vi "algo.configuration.vi"(11 "algo.data.in":T1={"next.state"=enum."Wait.for.Command", "saved.state"=enum."Wait.for.Command", "scratch"={"i"=0, "n"=0, "start.addr"=0, "first.call?"=FALSE, "j"=0, "o"=0, "k"=0, "p"=0, "just.write"=FALSE, "orderId "=0, "dir"=0}, "mode"=enum."Get.Symbol", "cmd.mem.watchlist"={"read.request"=FALSE, "read.addr"=0, "read.ready"=FALSE, "val.watchlist.read"={"symbol"=0, "buy.start.addr"=0, "buy.size"=0, "buy.slots"=0, "sell.start.addr"=0, "sell.size"=0, "sell.slots"=0, "min.ask"=0, "max.bid"=0}, "write.request"=FALSE, "write.addr"=0, "val.watchlist.write"={"symbol"=0, "buy.start.addr"=0, "buy.size"=0, "buy.slots"=0, "sell.start.addr"=0, "sell.size"=0, "sell.slots"=0, "min.ask"=0, "max.bid"=0}}, "cmd.mem.orders"={"read.addr"=0, "read.request"=FALSE, "read.ready"=FALSE, "write.addr"=0, "write.request"=FALSE, "read.data"={"OrderId"=0, "Price"=0, "Quantity"=0}, "write.data"={"OrderId"=0, "Price"=0, "Quantity"=0}}, "cmd.state"={"write.to.state"=FALSE, "val.state"=[0, 0, 0, 0]}, "cmd.debug"={"write.to.debug"=FALSE, "val.debug"=[0, 0]}, "stats"={"min.ask"=0, "max.bid"=0, "price"=0, "quantity"=0, "execution"=FALSE}, "orderbook.command"={"type"=enum."AddOrder", "side"=0, "orderId "=0, "quantity"=0, "symbol"=0, "price"=0, "executed.qty"=0, "canceled.qty"=0, "remaining.qty"=0, "seconds"=0, "nanoseconds"=0, "Add"=FALSE, "Edit"=FALSE, "Remove"=FALSE}, "time"={"last"=0, "since"=0}, "watchlist.size"=0, "active.watchlist"={"item"={"symbol"=0, "buy.start.addr"=0, "buy.size"=0, "buy.slots"=0, "sell.start.addr"=0, "sell.size"=0, "sell.slots"=0, "min.ask"=0, "max.bid"=0}, "index"=0}, "active.order"={"buy"=FALSE, "sell"=FALSE, "addr"=0, "size"=0, "slots"=0, "index"=0}} {"active.watchlist"."item"."symbol" format="%.0x"; "cmd.mem.orders"."write.data"."OrderId" format="%.0x"; "cmd.mem.orders"."read.data"."OrderId" format="%.0x"; "cmd.mem.watchlist"."val.watchlist.write"."symbol" format="%.0x"; "cmd.mem.watchlist"."val.watchlist.read"."symbol" format="%.0x"}) -> (0 "Ready.for.OrderBook.Command.Input":bool, 3 "algo.data.out":T1={"next.state"=enum."Wait.for.Command", "saved.state"=enum."Wait.for.Command", "scratch"={"i"=0, "n"=0, "start.addr"=0, "first.call?"=FALSE, "j"=0, "o"=0, "k"=0, "p"=0, "just.write"=FALSE, "orderId "=0, "dir"=0}, "mode"=enum."Get.Symbol", "cmd.mem.watchlist"={"read.request"=FALSE, "read.addr"=0, "read.ready"=FALSE, "val.watchlist.read"={"symbol"=0, "buy.start.addr"=0, "buy.size"=0, "buy.slots"=0, "sell.start.addr"=0, "sell.size"=0, "sell.slots"=0, "min.ask"=0, "max.bid"=0}, "write.request"=FALSE, "write.addr"=0, "val.watchlist.write"={"symbol"=0, "buy.start.addr"=0, "buy.size"=0, "buy.slots"=0, "sell.start.addr"=0, "sell.size"=0, "sell.slots"=0, "min.ask"=0, "max.bid"=0}}, "cmd.mem.orders"={"read.addr"=0, "read.request"=FALSE, "read.ready"=FALSE, "write.addr"=0, "write.request"=FALSE, "read.data"={"OrderId"=0, "Price"=0, "Quantity"=0}, "write.data"={"OrderId"=0, "Price"=0, "Quantity"=0}}, "cmd.state"={"write.to.state"=FALSE, "val.state"=[0, 0, 0, 0]}, "cmd.debug"={"write.to.debug"=FALSE, "val.debug"=[0, 0]}, "stats"={"min.ask"=0, "max.bid"=0, "price"=0, "quantity"=0, "execution"=FALSE}, "orderbook.command"={"type"=enum."AddOrder", "side"=0, "orderId "=0, "quantity"=0, "symbol"=0, "price"=0, "executed.qty"=0, "canceled.qty"=0, "remaining.qty"=0, "seconds"=0, "nanoseconds"=0, "Add"=FALSE, "Edit"=FALSE, "Remove"=FALSE}, "time"={"last"=0, "since"=0}, "watchlist.size"=0, "active.watchlist"={"item"={"symbol"=0, "buy.start.addr"=0, "buy.size"=0, "buy.slots"=0, "sell.start.addr"=0, "sell.size"=0, "sell.slots"=0, "min.ask"=0, "max.bid"=0}, "index"=0}, "active.order"={"buy"=FALSE, "sell"=FALSE, "addr"=0, "size"=0, "slots"=0, "index"=0}} {"active.watchlist"."item"."symbol" format="%.0x"; "cmd.mem.orders"."write.data"."OrderId" format="%.0x"; "cmd.mem.orders"."read.data"."OrderId" format="%.0x"; "cmd.mem.watchlist"."val.watchlist.write"."symbol" format="%.0x"; "cmd.mem.watchlist"."val.watchlist.read"."symbol" format="%.0x"})   [LabVIEW 2020]
uses:
  <vilib>/rvi/DataTransferAndStorage/Container/XNode/niFpgaContainer.xnode
  types/algo.states.ctl
  <vilib>/rvi/FIFO/Fifo_Resource/nirvififoEmulationRead.vi
  types/algo.scratch.ctl
  types/algo.mode.ctl
  types/algo.val.watchlist.ctl
  types/algo.cmd.mem.watchlist.ctl
  types/algo.cmd.mem.orders.ctl
  types/algo.val.state.ctl
  types/algo.cmd.state.ctl
  types/algo.val.debug.ctl
  types/algo.cmd.debug.ctl
  types/algo.stats.ctl
  common/orderbook.command.type.ctl
  common/orderbook.command.ctl
  types/algo.time.ctl
  algo.data.ctl
  types/algo.val.order.ctl
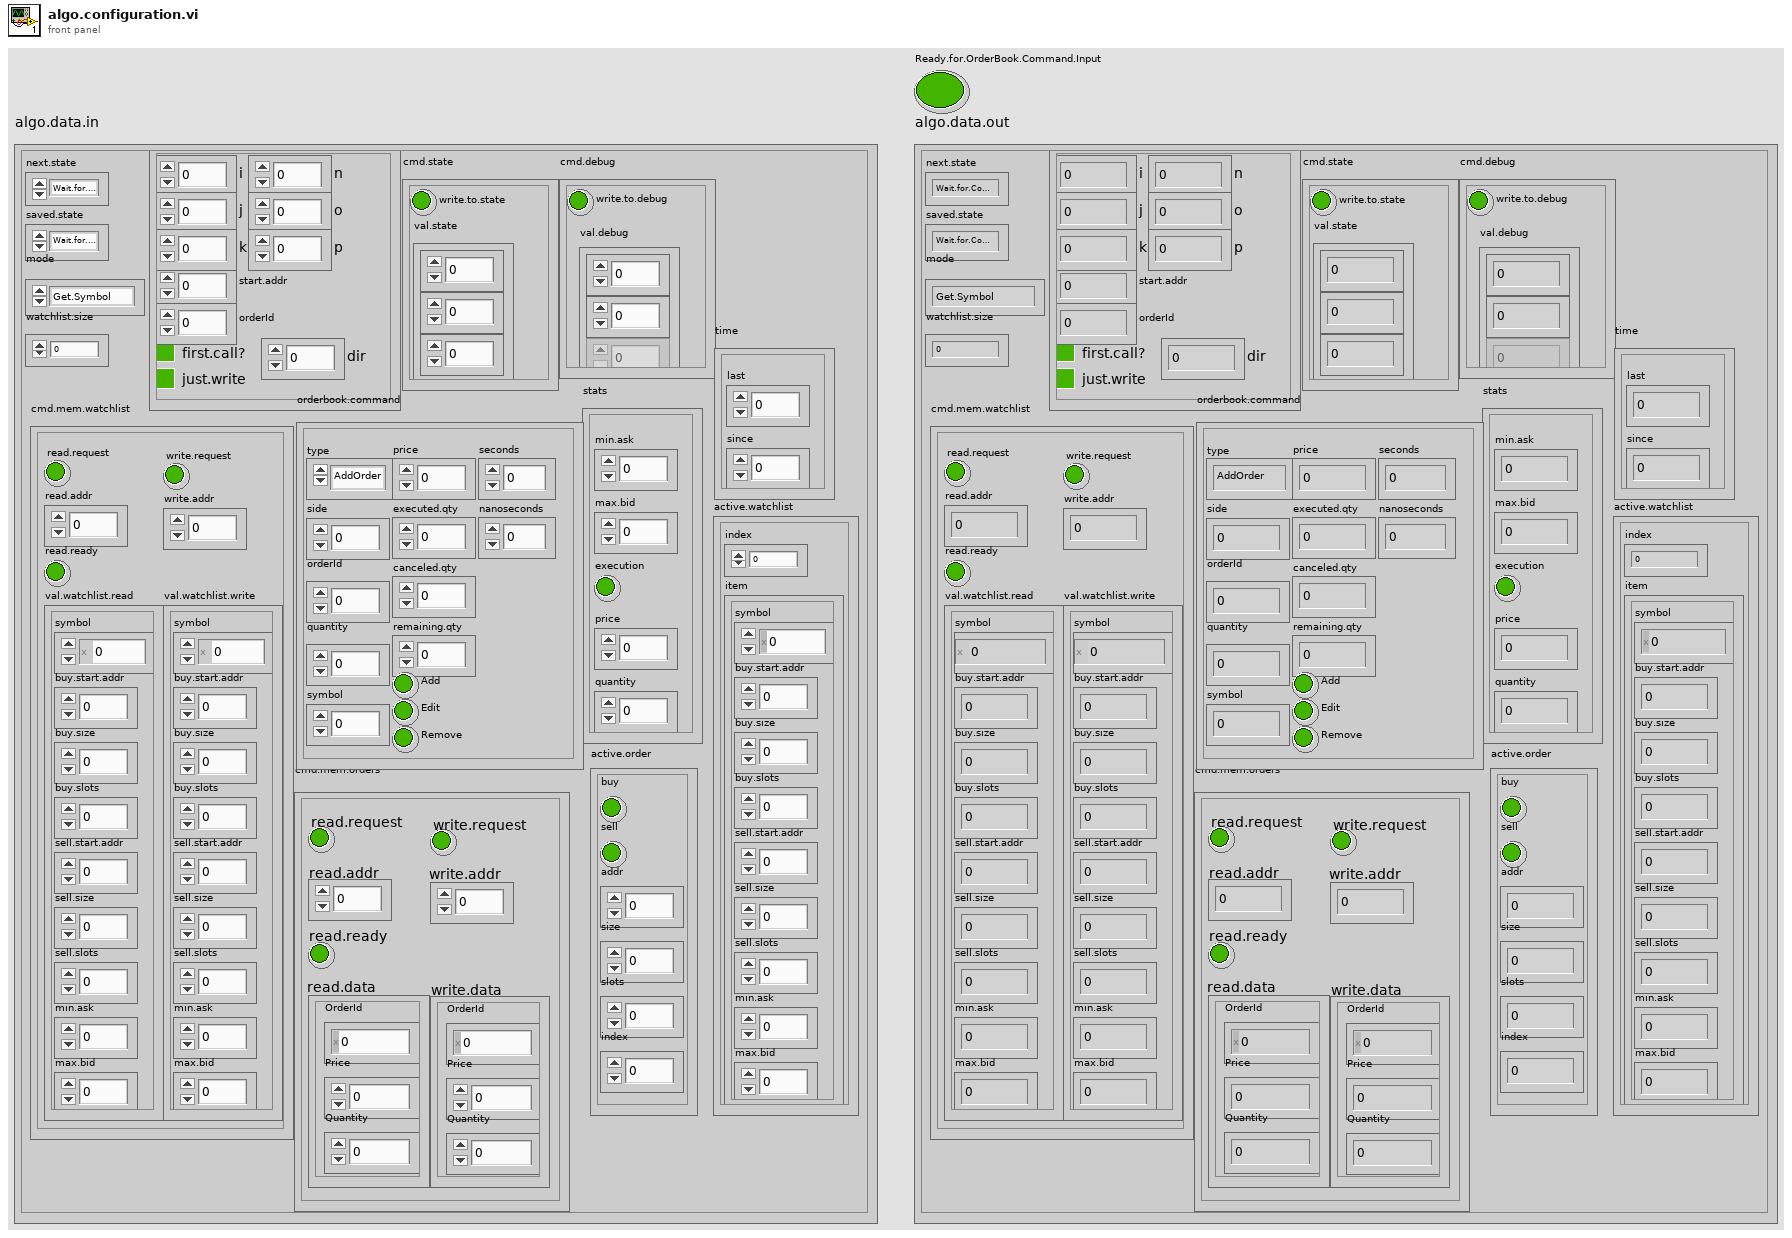
[diagram p1: front panel]
types:
  T1 = typedef "algo.data.ctl" = cluster{"next.state":T2, "saved.state":T2, "scratch":T3, "mode":T4, "cmd.mem.watchlist":T5, "cmd.mem.orders":T7, "cmd.state":T9, "cmd.debug":T11, "stats":T13, "orderbook.command":T14, "time":T16, "watchlist.size":u64, "active.watchlist":cluster{"item":T6, "index":u64}, "active.order":cluster{"buy":bool, "sell":bool, "addr":i16, "size":i16, "slots":i16, "index":i16}}
  T2 = typedef "algo.states.ctl" = enum16{"Noop", "Reset", "Configuration", "Debug", "Get.State", "Wait.for.Command", "Process.Command"}
  T3 = typedef "algo.scratch.ctl" = cluster{"i":u64, "n":u64, "start.addr":u16, "first.call?":bool, "j":u64, "o":u64, "k":u64, "p":u64, "just.write":bool, "orderId ":u64, "dir":i8}
  T4 = typedef "algo.mode.ctl" = enum16{"watchlist.iter", "order.buy.iter", "order.sell.iter", "Get.Symbol", "Search", "Shift"}
  T5 = typedef "algo.cmd.mem.watchlist.ctl" = cluster{"read.request":bool, "read.addr":u16, "read.ready":bool, "val.watchlist.read":T6, "write.request":bool, "write.addr":u16, "val.watchlist.write":T6}
  T6 = typedef "algo.val.watchlist.ctl" = cluster{"symbol":u64, "buy.start.addr":u16, "buy.size":u16, "buy.slots":u16, "sell.start.addr":u16, "sell.size":u16, "sell.slots":u16, "min.ask":u64, "max.bid":u64}
  T7 = typedef "algo.cmd.mem.orders.ctl" = cluster{"read.addr":u16, "read.request":bool, "read.ready":bool, "write.addr":u16, "write.request":bool, "read.data":T8, "write.data":T8}
  T8 = typedef "algo.val.order.ctl" = cluster{"OrderId":u64, "Price":u64, "Quantity":u32}
  T9 = typedef "algo.cmd.state.ctl" = cluster{"write.to.state":bool, "val.state":T10}
  T10 = typedef "algo.val.state.ctl" = u64[]
  T11 = typedef "algo.cmd.debug.ctl" = cluster{"write.to.debug":bool, "val.debug":T12}
  T12 = typedef "algo.val.debug.ctl" = u64[]
  T13 = typedef "algo.stats.ctl" = cluster{"min.ask":u32, "max.bid":u32, "price":u32, "quantity":u32, "execution":bool}
  T14 = typedef "orderbook.command.ctl" = cluster{"type":T15, "side":u8, "orderId ":u64, "quantity":u32, "symbol":u64, "price":u64, "executed.qty":u32, "canceled.qty":u32, "remaining.qty":u32, "seconds":u64, "nanoseconds":u64, "Add":bool, "Edit":bool, "Remove":bool}
  T15 = typedef "orderbook.command.type.ctl" = enum8{"Time", "AddOrder", "OrderExecuted", "OrderExecutedAtPrice", "ReduceSize", "ModifyOrder", "DeleteOrder", "Get.Everything", "Get.All.Orders", "Get.Top"}
  T16 = typedef "algo.time.ctl" = cluster{"last":u32, "since":u32}
  T17 = cluster{"symbol":u64, "buy.start.addr":u16, "buy.size":u16, "buy.slots":u16, "sell.start.addr":u16, "sell.size":u16, "sell.slots":u16, "min.ask":u64, "max.bid":u64}
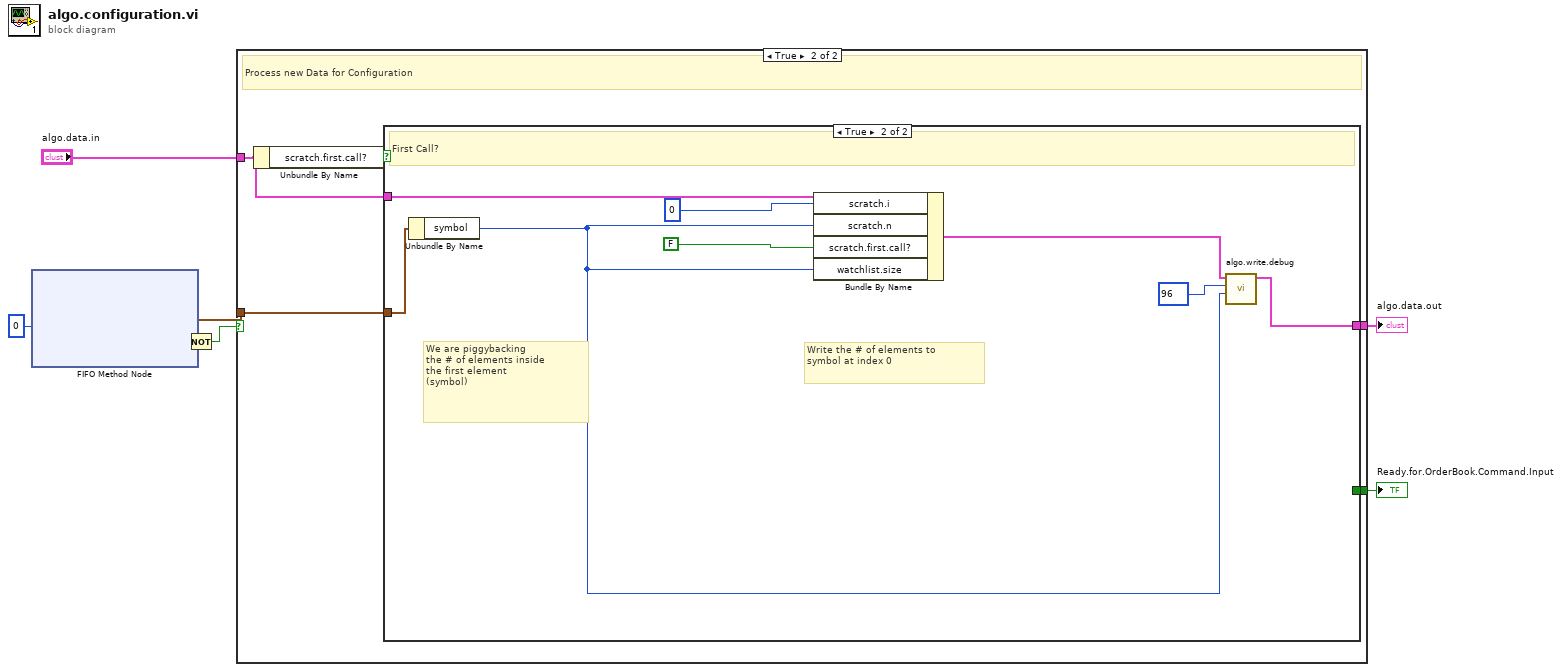
[diagram p0: block diagram]
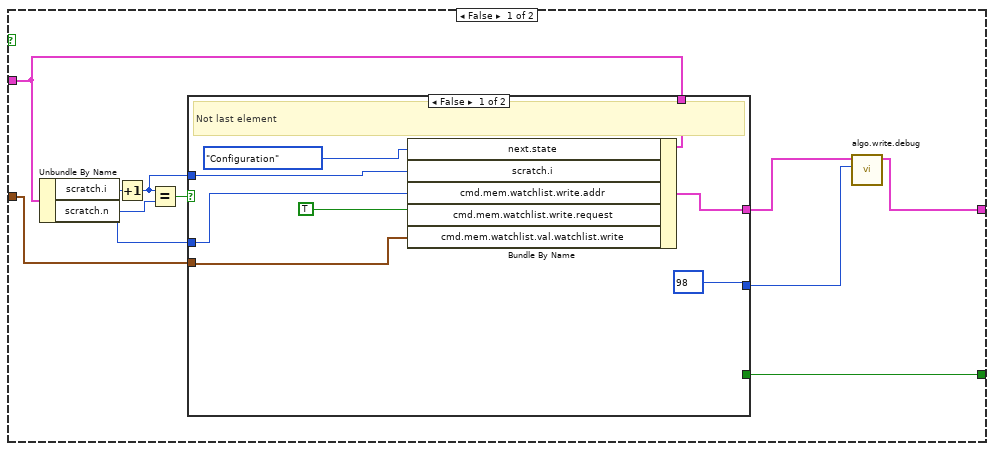
[diagram p3: hidden frame]
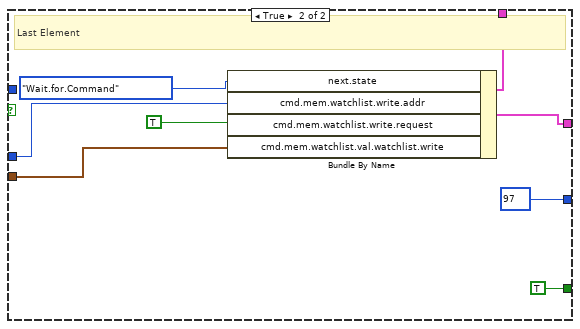
[diagram p4: hidden frame]
diagram:
  n1 = xnode ("FIFO Method Node")("Timeout"=0) -> ("Element"=w5:T17, "Timed Out?"=w3:bool)  [unwired: 1 in, 1 out]
  n2 = Not(x=w3) -> (.not. x?=w1:bool)
  n3 = case shown="True" w1 {
    tunnel: [w8 w10] -> w7
    tunnel: "algo.data.in" -> [w8 w11]
    tunnel: w5 -> [_ w12]
    tunnel: [_ w9] -> w4
    frame False {
      # "No new data, noop wait for new data"
    }
    frame True {
      # "Process new Data for Configuration"
      n4 = Unbundle By Name(w11) -> ("scratch.first.call?"=w13:bool)
      n5 = case shown="True" w13 {
        tunnel: w12 -> [w15 w42]
        tunnel: w11 -> [w23 w47]
        tunnel: [w17 w44] -> w10
        tunnel: [w19 _] -> w9
        frame False {
          n6 = Unbundle By Name(w23) -> ("scratch.i"=w20:u64, "scratch.n"=w22:u64)
          n7 = Increment(x=w20) -> (x+1=w16:u64)
          n8 = Equal?(x=w16, y=w22) -> (x = y?=w21:bool)
          n9 = case shown="False" w21 {
            tunnel: [w31 w39] -> w18
            tunnel: w23 -> [w27 w38]
            tunnel: w20 -> [w28 w36]
            tunnel: w16 -> [w29 _]
            tunnel: [_ TRUE] -> w19
            tunnel: w15 -> [w25 w33]
            tunnel: [u64 98 ("Dbg.Val.1") u64 97 ("Dbg.Val.1")] -> w14
            frame False {
              # "Not last element"
              n10 = Bundle By Name(cluster=w27, "next.state"=algo.states."Configuration", "scratch.i"=w29, "cmd.mem.watchlist.write.addr"=w28, "cmd.mem.watchlist.write.request"=TRUE, "cmd.mem.watchlist.val.watchlist.write"=w25) -> (w31:T1)
            }
            frame True {
              # "Last Element"
              n11 = Bundle By Name(cluster=w38, "next.state"=algo.states."Wait.for.Command", "cmd.mem.watchlist.write.addr"=w36, "cmd.mem.watchlist.write.request"=TRUE, "cmd.mem.watchlist.val.watchlist.write"=w33) -> (w39:T1)
            }
          }
          n12 = call "algo.write.debug.vi"("dbg.val.1"=w14, "algo.data.in"=w18) -> ("algo.data.out"=w17:T1)  [unwired: 9 in]
        }
        frame True {
          # "Write the # of elements to\nsymbol at index 0"
          # "We are piggybacking\nthe # of elements inside\nthe first element\n(symbol)"
          # "First Call?"
          n13 = Unbundle By Name(w42) -> ("symbol"=w40:u64)
          n14 = Bundle By Name(cluster=w47, "scratch.i"=u64 0, "scratch.n"=w40, "scratch.first.call?"=FALSE, "watchlist.size"=w40) -> (w45:T1)
          n15 = call "algo.write.debug.vi"("dbg.val.2"=w40, "dbg.val.1"=u64 96 ("Dbg.Val.1"), "algo.data.in"=w45) -> ("algo.data.out"=w44:T1)  [unwired: 8 in]
        }
      }
    }
  }
  "Ready.for.OrderBook.Command.Input" <- w4
  "algo.data.out" <- w7
